vi "Model 3566-Sampling.vi"(8 "error in":errorcluster, 10 "Sampling":enum16{"SLOW", "MEDIUM", "FAST"}(ring), 11 "Model 3566 Setting In":T1) -> (0 "error out":errorcluster, 3 "Model 3566 Setting Out":T1)   [LabVIEW 2018]
uses:
  Data Def/Model 3566-Setting.ctl
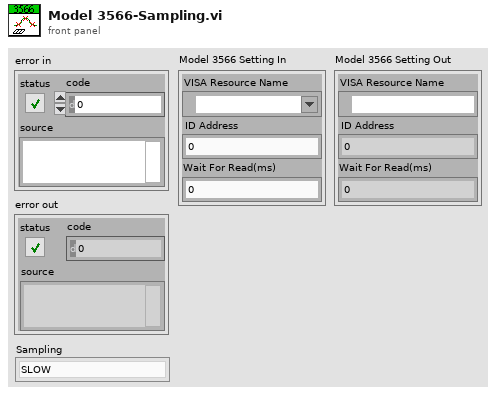
[diagram p1: front panel]
types:
  T1 = typedef "Model 3566-Setting.ctl" = cluster{"VISA Resource Name":refnum<visa-resource-name>, "ID Address":u8, "Wait For Read(ms)":u32}
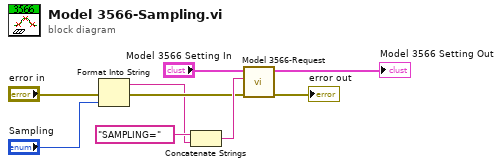
[diagram p0: block diagram]
diagram:
  n1 = Format Into String(error in="error in", "Sampling") -> (resulting string=w4:string, error out=w6:errorcluster)  [unwired: 2 in]
  n2 = Concatenate Strings("SAMPLING=" ("write buffer"), w4) -> (w7:string)
  n3 = call "Model 3566-Request.vi"("error in"=w6, "Command"=w7, "Model 3566 Setting In"="Model 3566 Setting In") -> ("error out"=→"error out":errorcluster, "Model 3566 Setting Out"=→"Model 3566 Setting Out":T1)  [unwired: 6 in, 1 out]
